vi "LogViewer.vi"(7 "Current Module(\"\" to generate an ID)":string="logViewer") -> ()   [LabVIEW 2017, in "DebugConsole.lvlib"]
uses:
  DebugConsole.lvlib
  Utility/_support/Periodic String Filter Level.ctl
  Utility/Periodic String Filter Setting.ctl
  <vilib>/addons/_JKI Toolkits/State Machine/_JKI_lib_State_Machine.llb/Parse State Queue__JKI_lib_State_Machine.vi
  _csmlite/_Engine.vi
  _csmlite/_PassAllowedMessage - MsgList.vi
  Communicable State Machine.lvlib
  _Shared/CSM Shared.lvlib
  _Support/csm-tool-support.lvlib
  _csmHelper/API with lvcsm Support/CSM-Helper API with lvcsm Support.lvlib
  addons/Logger/CSM File Logger.lvlib
  _ui/csm-ui-support.lvlib
  _csmlite/_csmlite.lvlib
panel:
  out "Error(#)":i64 caption="Error(#):"
  in  "Record.Stop":bool
  in  "Record.Start":bool
  in  "Clear":bool
  in  "BackTop":bool
  in  "Toolbar.History Length(char)":i32=50000 caption="History(char)" min=1000 max=100000000 step=1
  in  "Peroid Logs":bool
  in  "Tab":T1(tab)
  out "State History":string
  out "Error History":string
  out "Userlog History":string
  out "LogInQ":i32 caption="LogInQ:"
  out "log handling Speed(#/s)":dbl caption="log handling Speed(#/s):"
  out "LogInQ change(#/s)":dbl caption="LogInQ change(#/s):"
  out "Level":T2 caption="Level:"
  in  "Stop":bool
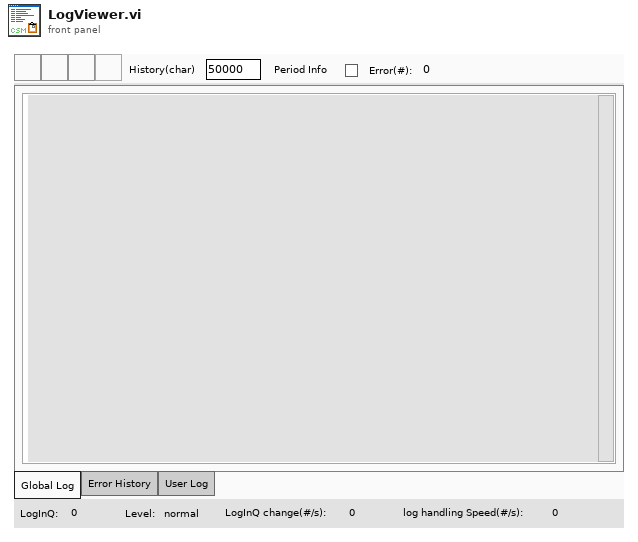
[diagram p1: front panel]
types:
  T1 = enum32{"Global Log", "Error History", "User Log"}
  T2 = typedef "Communicable State Machine.lvlib/Periodic String Filter Level.ctl" = enum16{"normal", "L1", "L2", "L3", "L4"}
  T3 = typedef "Communicable State Machine.lvlib/Periodic String Filter Setting.ctl" = cluster{"threashold(#/s)":dbl, "Check Peroid(s)":dbl}
  T4 = typedef "Communicable State Machine.lvlib/_CSM_GlobalLog_MSG.ctl" = cluster{"Name (\"\" to Use UUID)":string, "Current State":string, "Arguments":string, "Source Message":T5, "Source Module":string, "Complete(T)/Start(F)":bool, "LogType":T6, "Time Stamp":timestamp}
  T5 = typedef "Communicable State Machine.lvlib/_CSM_Response Source Message.ctl" = cluster{"‘State":string, "’Arguments":string, "’Error":errorcluster}
  T6 = typedef "Communicable State Machine.lvlib/_CSM_GlobalLog_MSG_TYPE.ctl" = enum16{"User Log", "State Change", "Status", "Interrupt", "Register", "Unregister", "Error Log", "Module Created", "Module Destroyed", "Async Message", "No-Rep Async Message", "Sync Message"}
  T7 = enum32{"Invalid", "Standard", "Closed", "Hidden", "Minimized", "Maximized"}
  T8 = enum32{"invalid app kind", "Development System", "Run Time System", "Student Edition", "Embedded LabVIEW", "Evaluation", "Custom"}
  T9 = typedef "LVPoint32TypeDef.ctl" = cluster{"Horizontal":i32, "Vertical":i32}
  T10 = cluster{"Shift":bool, "Ctrl":bool, "Alt":bool, "Cmd":bool, "Opt":bool}
  T11 = cluster{"Core":cluster{"Current VI Reference":refnum<vi>, "Close Panel on Exit?":bool}, "Toolbar.Advance":refnum<vi>[], "LoggerWatchDogQueue":refnum<queue>, "LogFile":path}
  T12 = cluster{"Current VI Reference":refnum<vi>, "Close Panel on Exit?":bool}
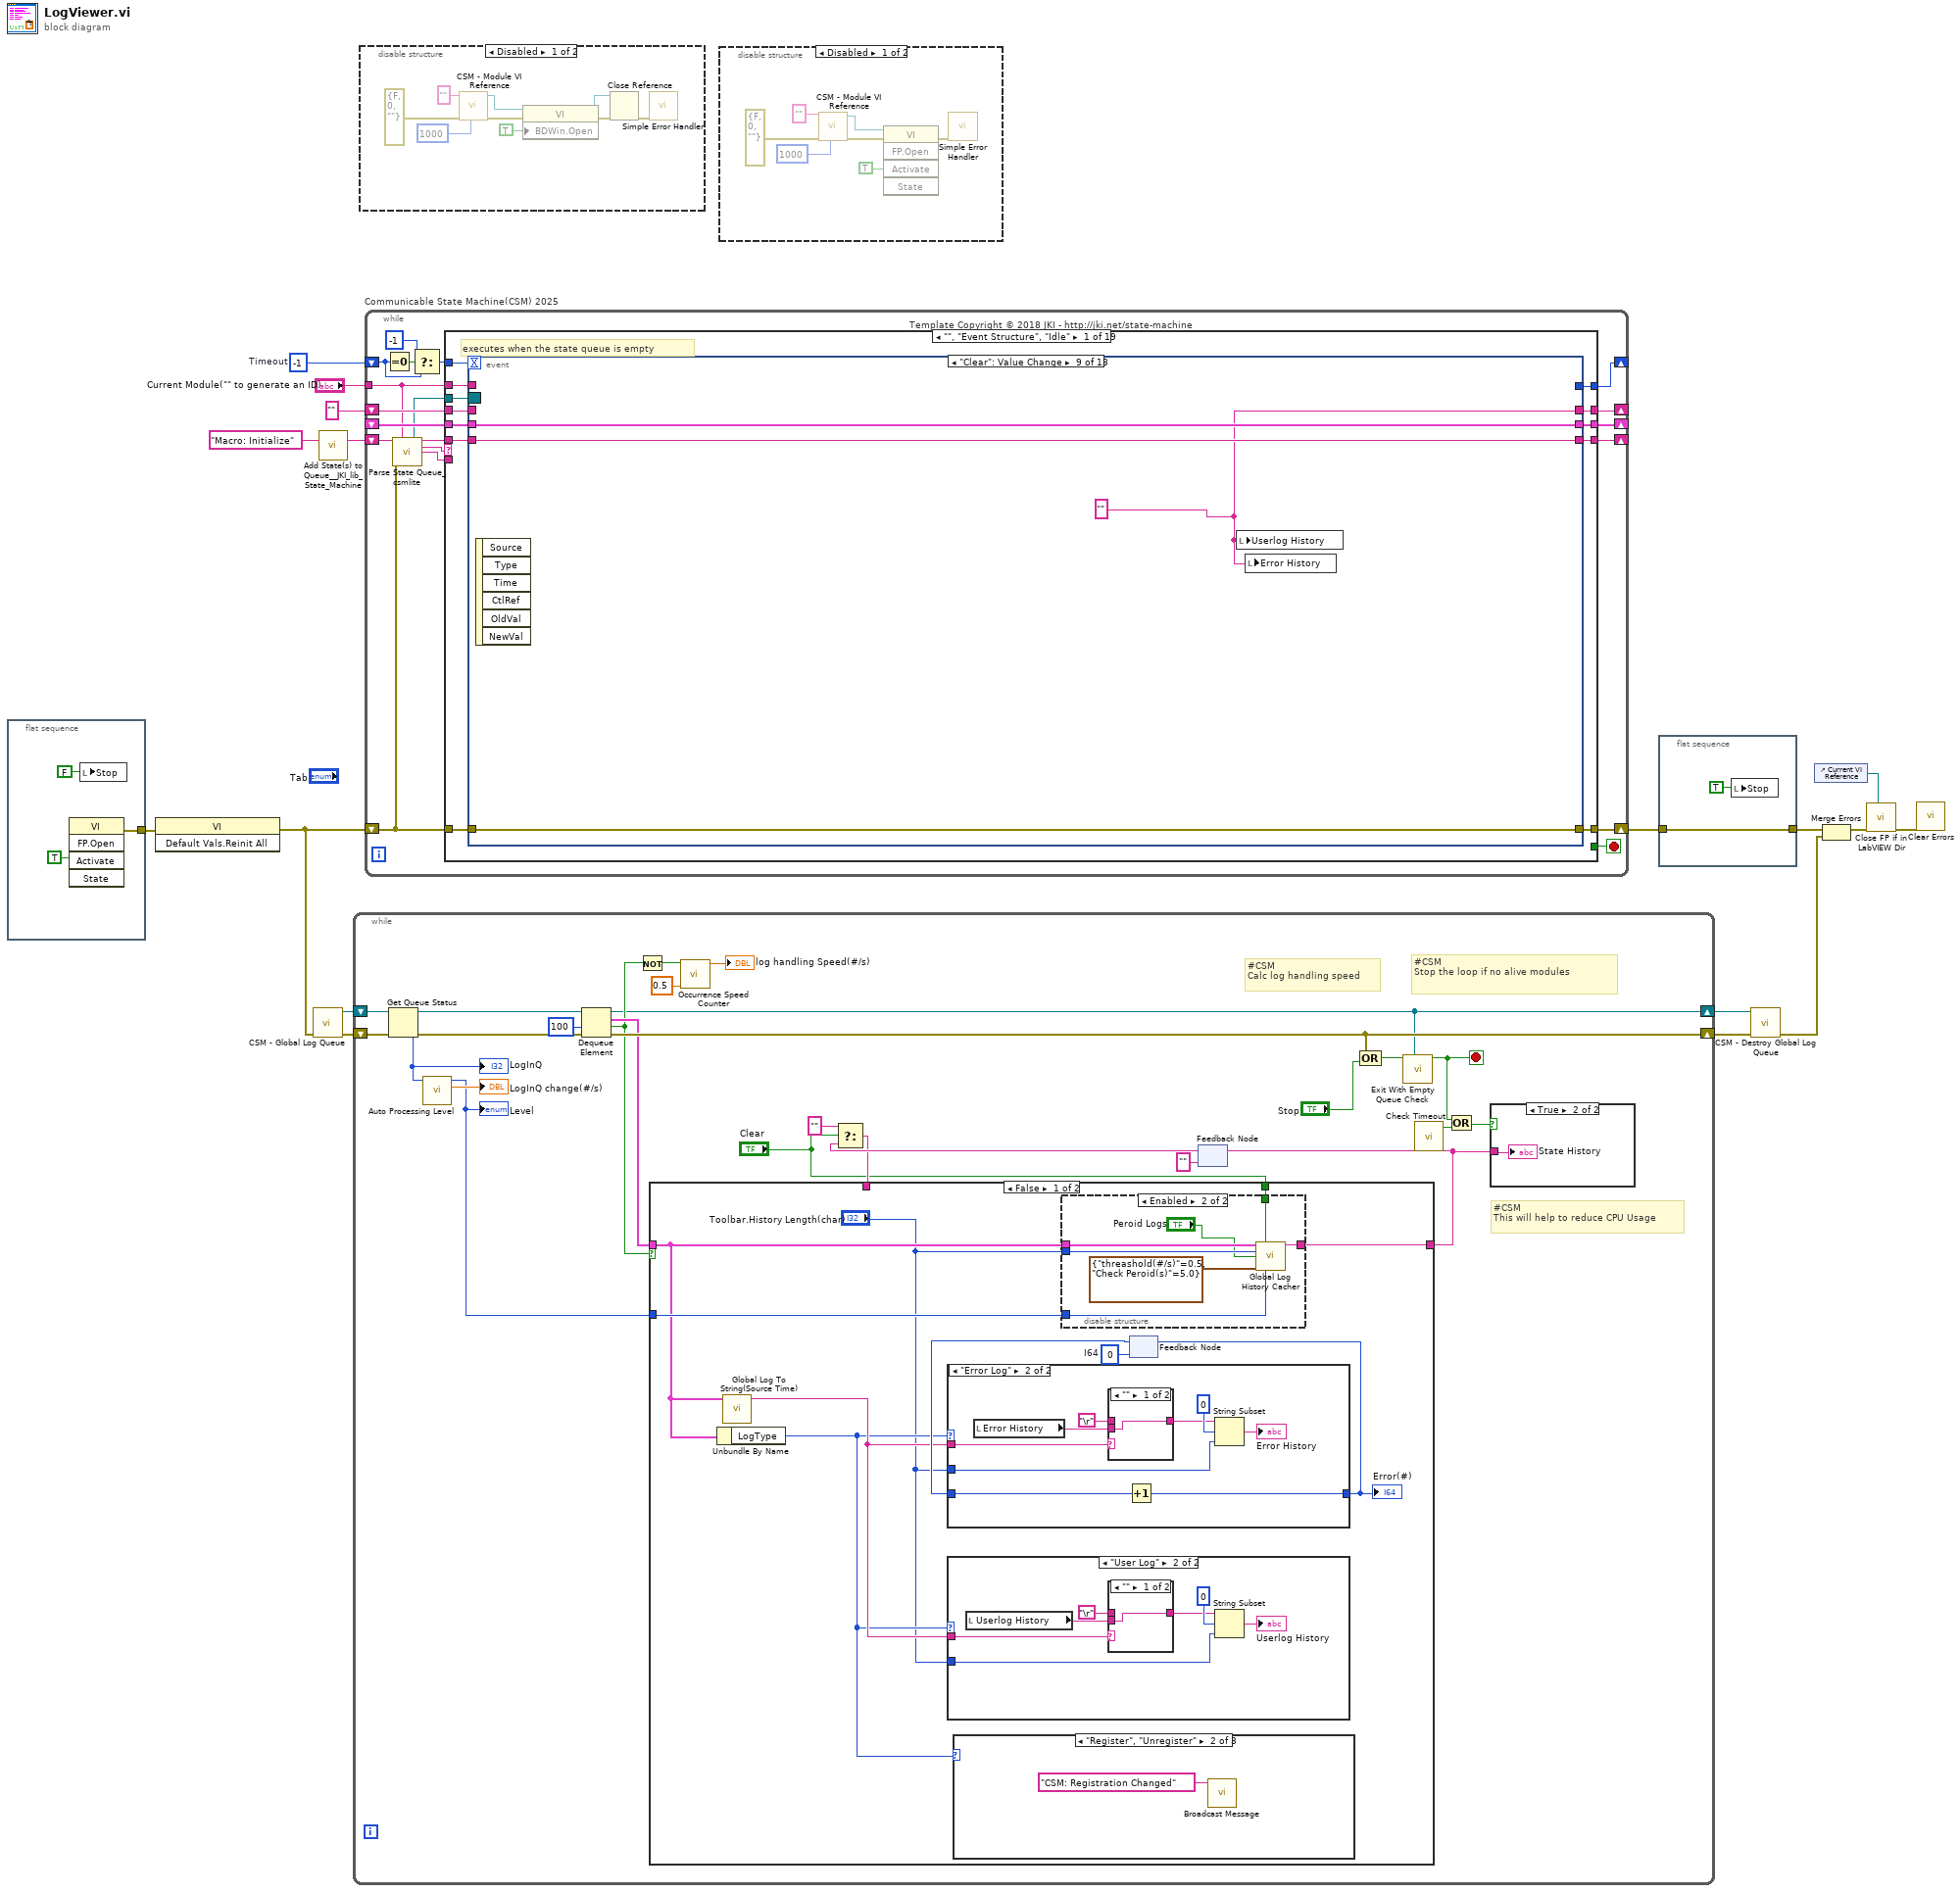
[diagram p0: block diagram]
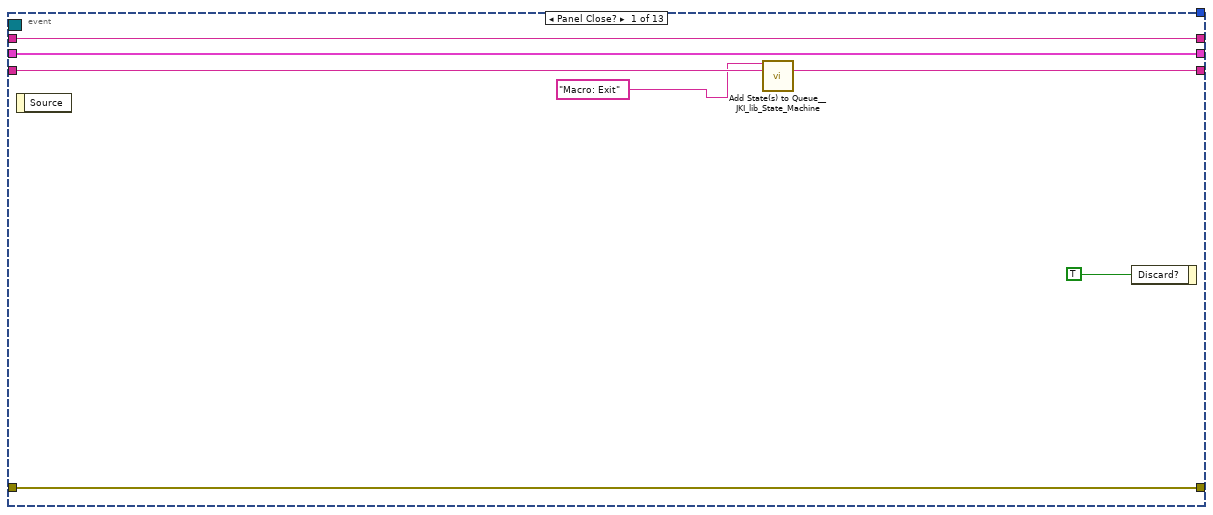
[diagram p4: hidden frame]
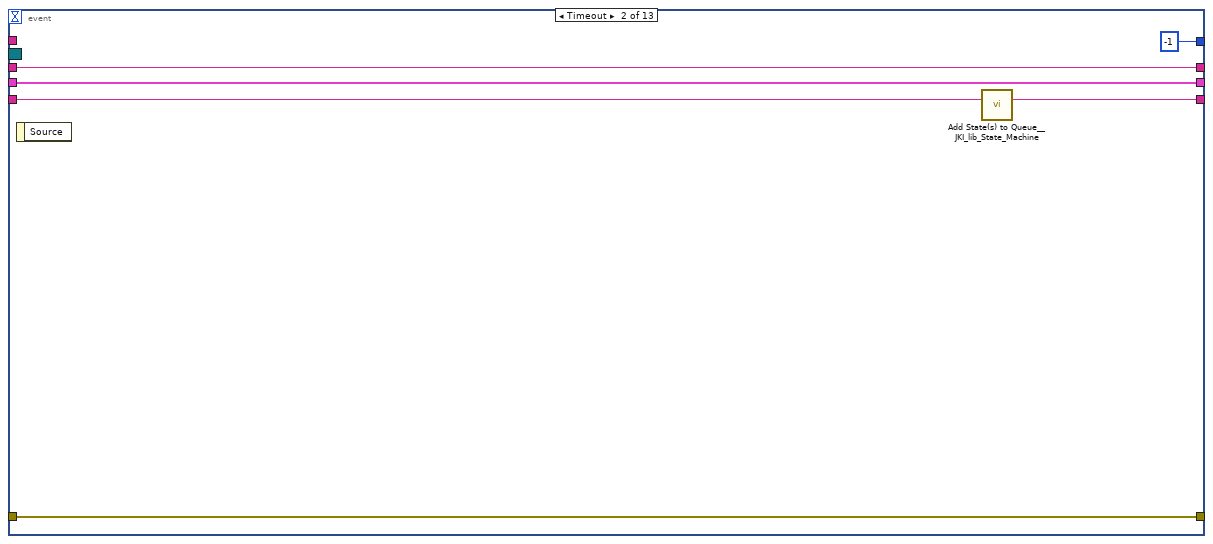
[diagram p5: hidden frame]
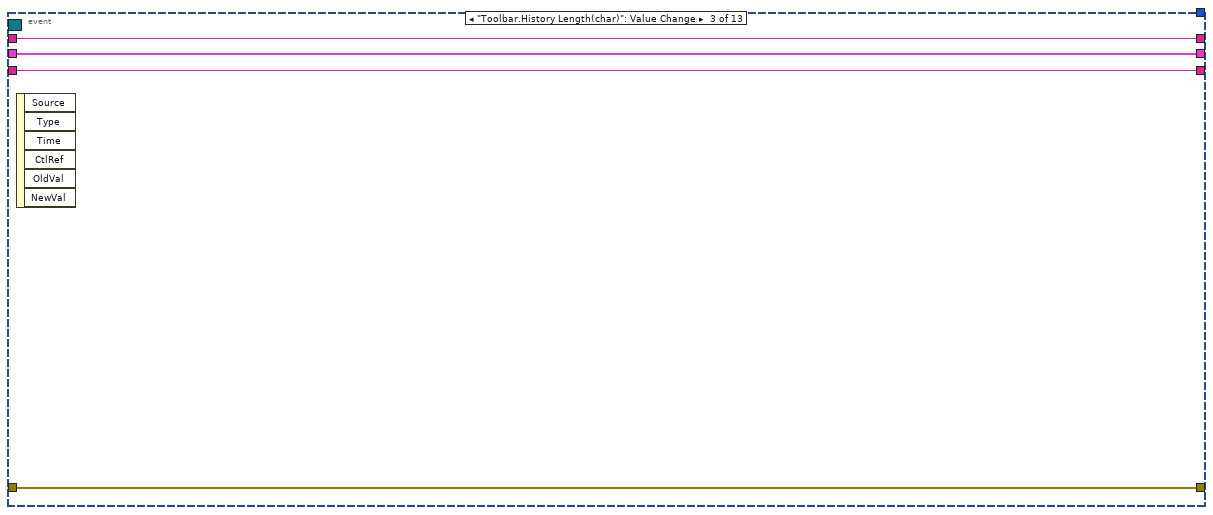
[diagram p6: hidden frame]
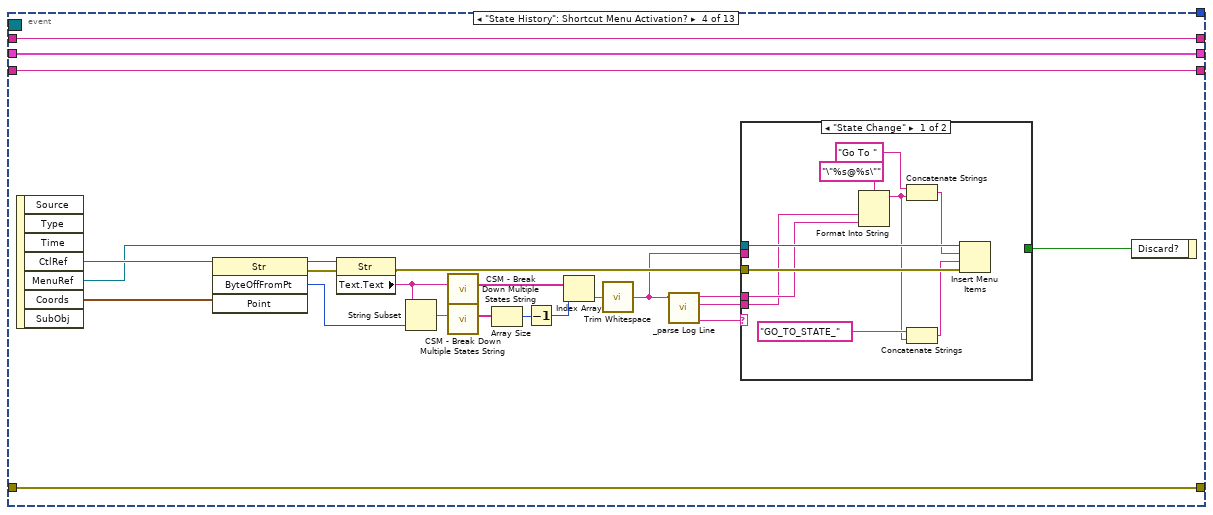
[diagram p7: hidden frame]
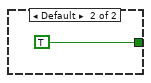
[diagram p8: hidden frame]
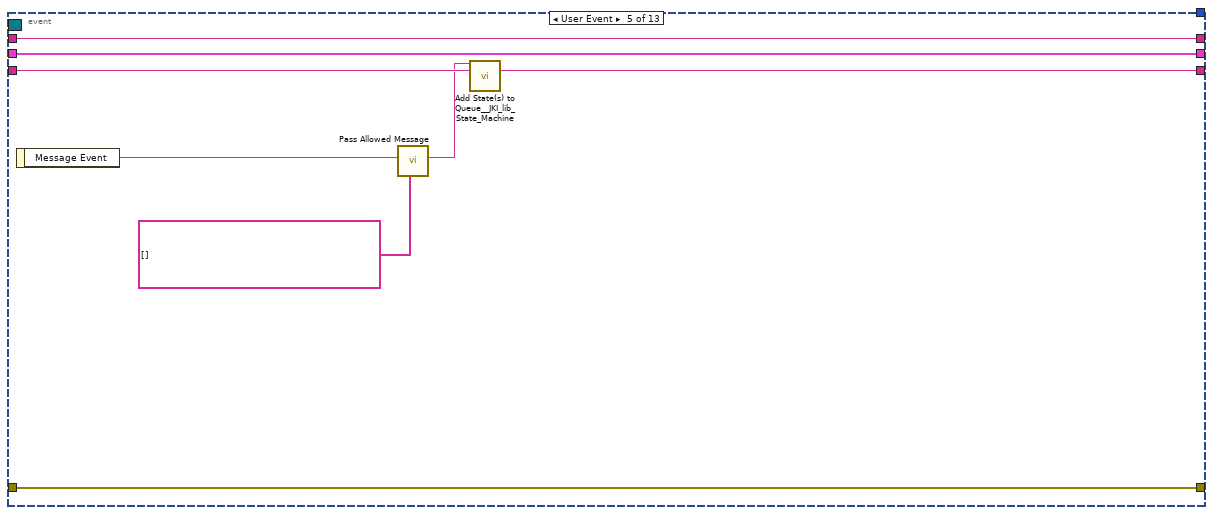
[diagram p9: hidden frame]
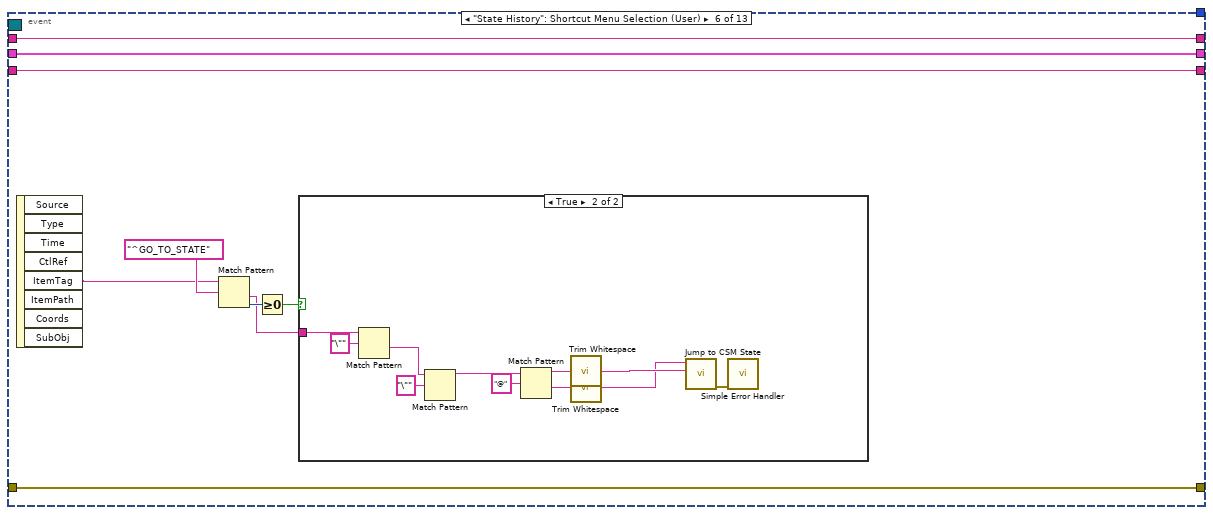
[diagram p10: hidden frame]
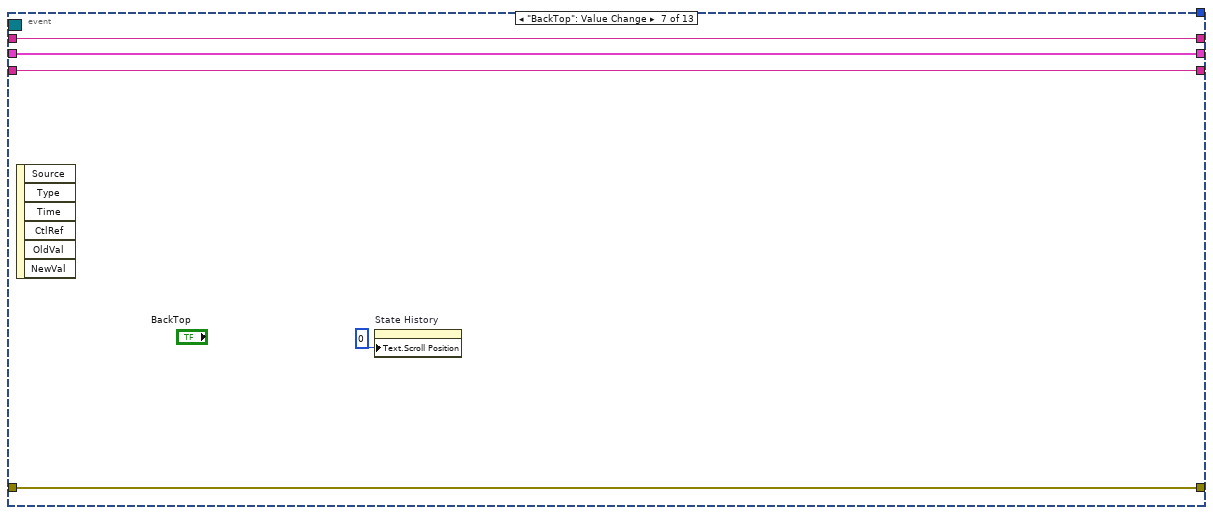
[diagram p12: hidden frame]
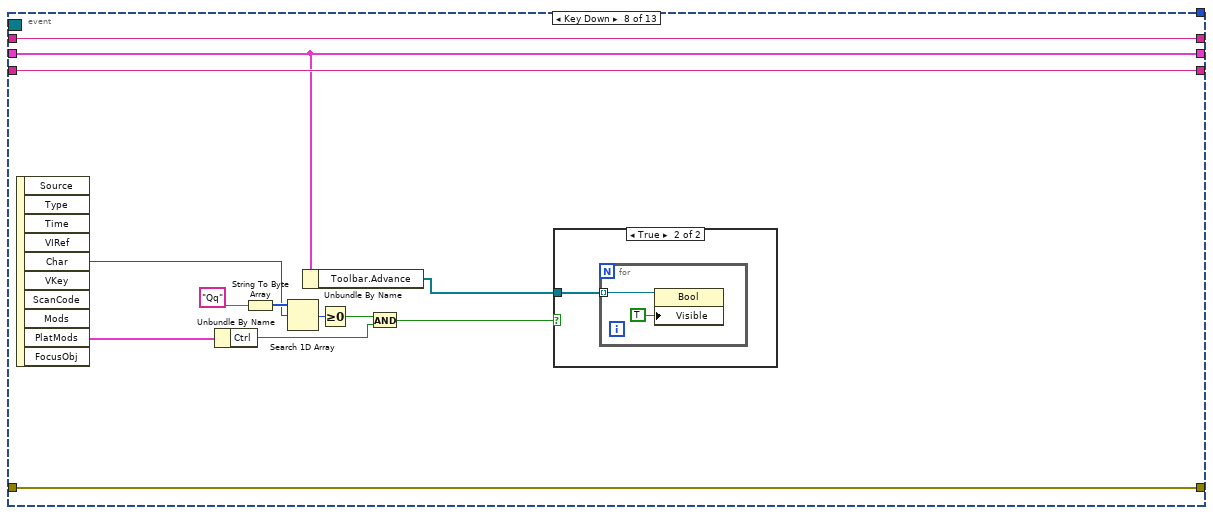
[diagram p13: hidden frame]
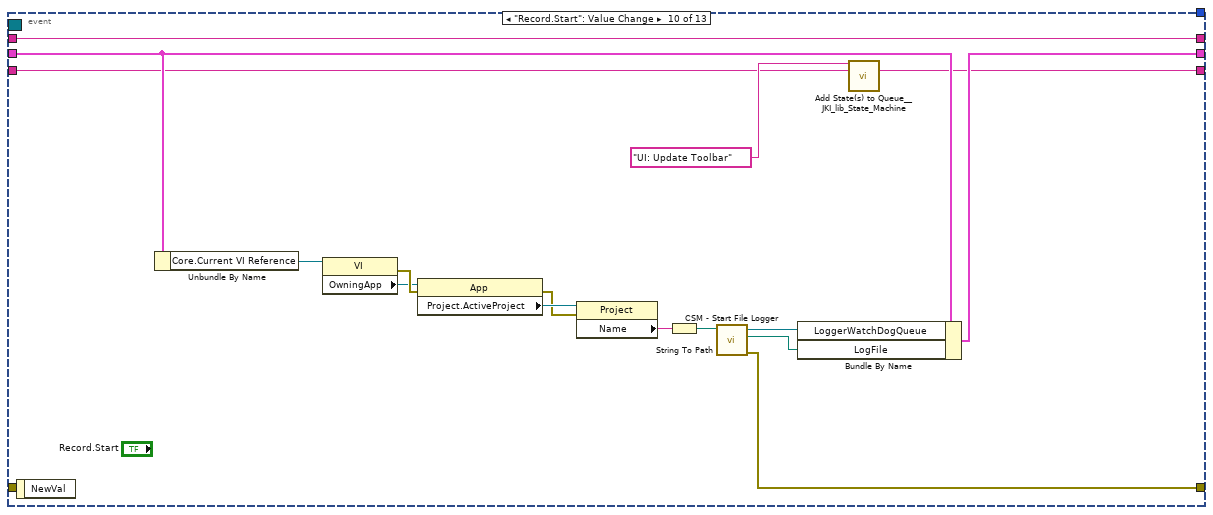
[diagram p15: hidden frame]
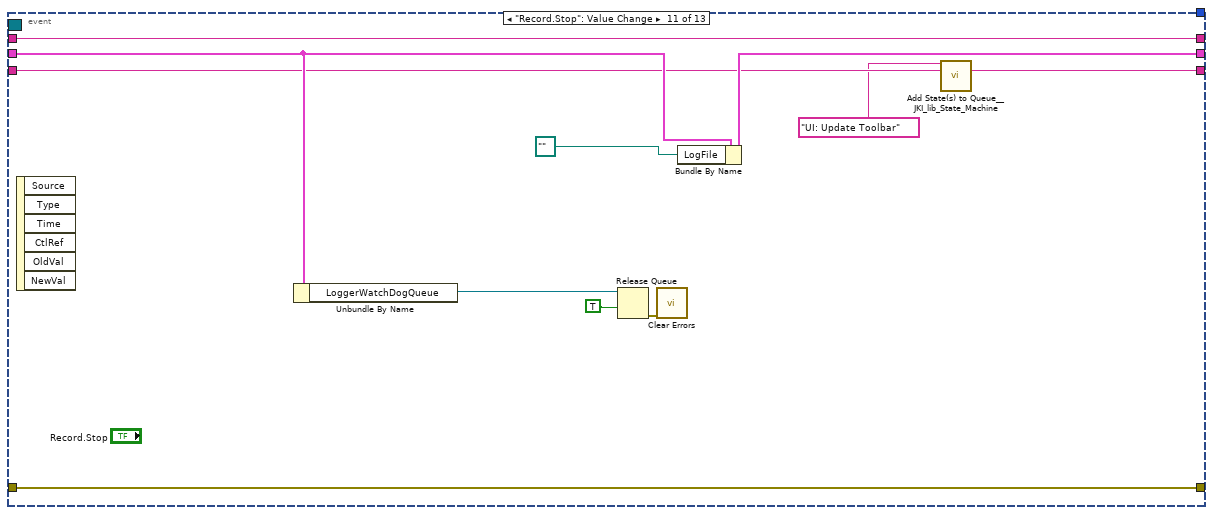
[diagram p16: hidden frame]
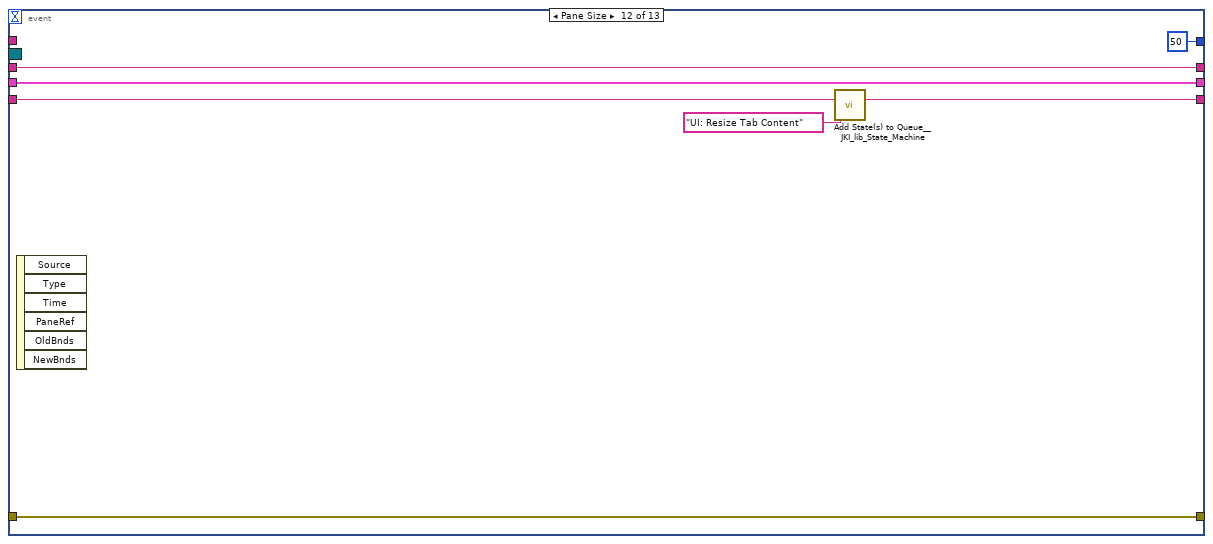
[diagram p17: hidden frame]
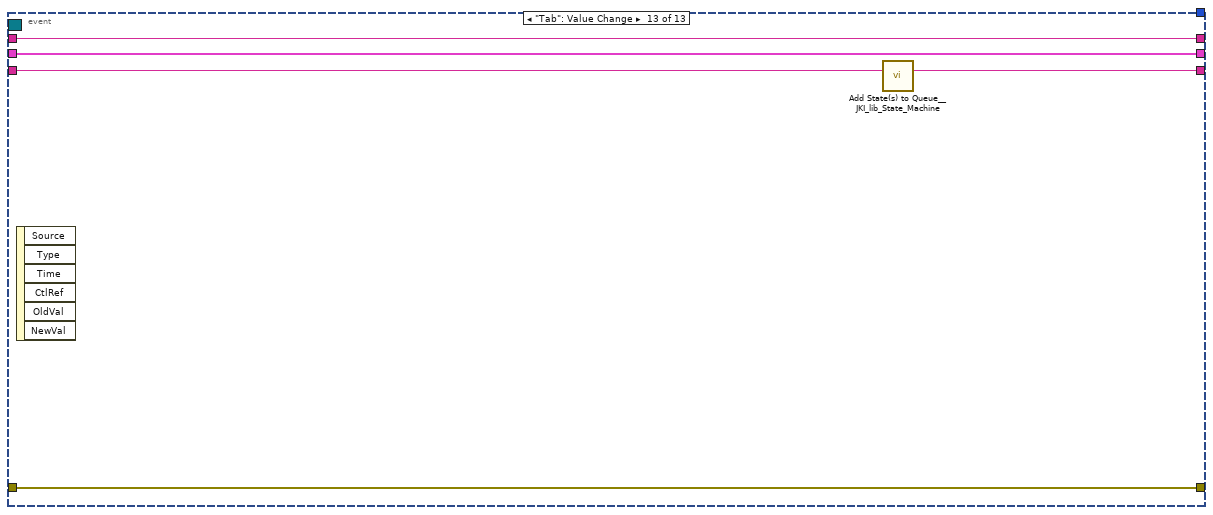
[diagram p18: hidden frame]
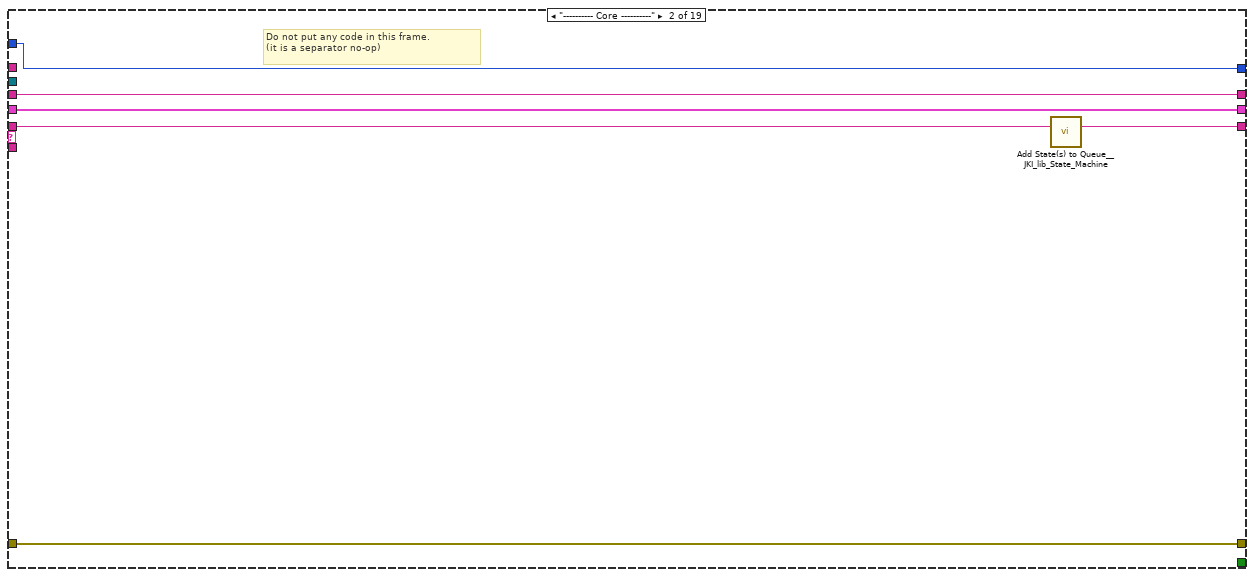
[diagram p19: hidden frame]
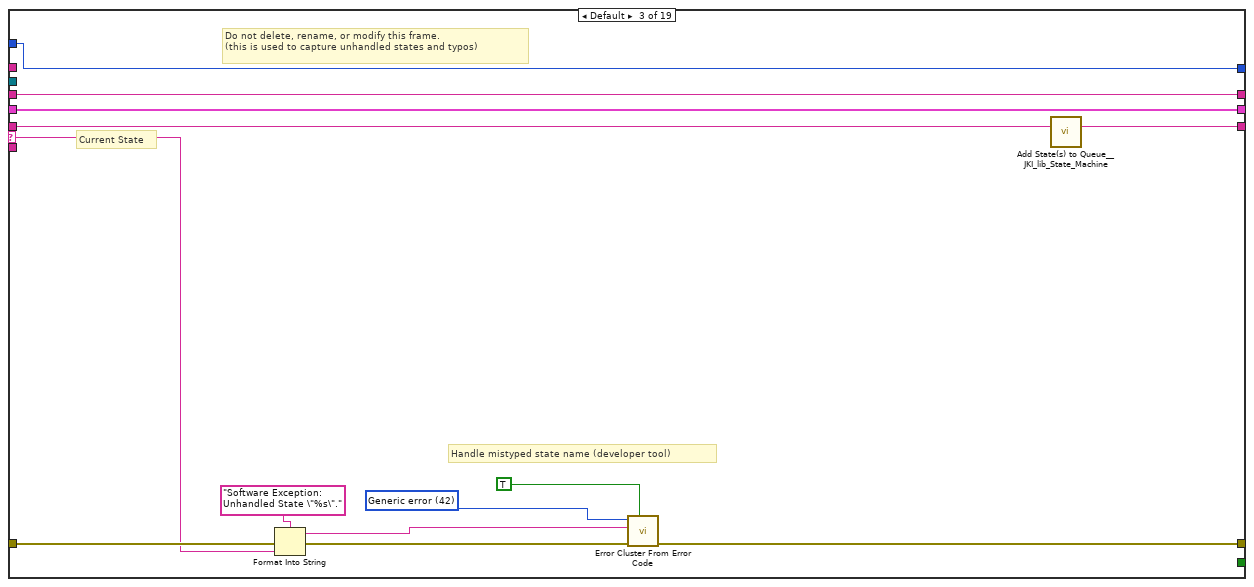
[diagram p20: hidden frame]
diagram:
  w10 = -1  # Timeout
  n1 = flat-sequence {
    tunnel: [w18] -> w6
    frame #0 {
      n2 = invoke class="VI" method="FP.Open"("Activate"=TRUE ("Activate?")) -> (error out=w18:errorcluster)  [unwired: 4 in, 4 out]
      n3 = local write "Stop"(FALSE ("Stop")) -> ()
    }
  }
  n4 = invoke class="VI" method="Default Vals.Reinit All"(error in=w6) -> (error out=w1:errorcluster)  [unwired: 2 in, 2 out]
  n5 = call "CSM - Global Log Queue.vi"("Error In"=w1) -> ("error out"=w16:errorcluster, "Global Log Queue"=w14:refnum<queue>)  [unwired: 9 in]
  n6 = call <vilib>:"Add State(s) to Queue__JKI_lib_State_Machine.vi"("State(s) in (\"\")"="Macro: Initialize") -> ("States Out"=w13:string)  [unwired: 14 in]
  n7 = while {
    shift-right: [w45] -> w17
    shift-left: w16 -> [w42]
    shift-right: [w33] -> w15
    shift-left: w14 -> [w46]
    stop <- w26 stop-if-true
    # "#CSM\nCalc log handling speed"
    # "#CSM\nStop the loop if no alive modules"
    # "#CSM\nThis will help to reduce CPU Usage"
    n8 = Get Queue Status(queue=w46, error in (no error)=w42) -> (queue out=w44:refnum<queue>, error out=w43:errorcluster, # elements in queue=w29:i32)  [unwired: 1 in, 5 out]
    "LogInQ" <- w29
    n9 = call "Auto Processing Level.vi"("#Left In Q"=w29) -> ("LogInQ Changing Speed (#/s)"=→"LogInQ change(#/s)":dbl, "Level"=w28:T2)  [unwired: 8 in, 1 out]
    "Level" <- w28
    n10 = Dequeue Element(queue=w44, timeout in ms (-1)=100, error in (no error)=w43) -> (queue out=w33:refnum<queue>, element=w41:T4, timed out?=w35:bool, error out=w45:errorcluster)
    n11 = Not(x=w35) -> (.not. x?=w34:bool)
    n12 = call "Occurrence Speed Counter.vi"("Period (0.1s)"=0.5, "Occured? (T)"=w34) -> ("Speed (#/s)"=→"log handling Speed(#/s)":dbl)  [unwired: 7 in, 2 out]
    n13 = feedback #1("" ("String Cache")) -> (w24:string)
    n14 = Select(t="", s="Clear", f=w24) -> (s? t:f=w23:string)
    n15 = case shown="False" w35 {
      tunnel: w41 -> [w54 _]
      tunnel: [w56 w96] -> w38
      tunnel: w23 -> [_ w96]
      tunnel: w28 -> [w55 _]
      tunnel: "Clear" -> [w47 _]
      frame False {
        w52 = i64 0  # I64
        n16 = Unbundle By Name(w54) -> ("LogType"=w49:T6)
        n17 = call "Global Log To String(Source Time).vi"("Log"=w54) -> ("Log String"=w50:string)  [unwired: 9 in]
        n18 = case shown="\"User Log\"" w49 {
          tunnel: w50 -> [_ w58]
          tunnel: "Toolbar.History Length(char)" -> [_ w57]
          frame Default {
          }
          frame "User Log" {
            n19 = local read "Userlog History"() -> (w62:string)
            n20 = case shown="\"\"" w58 {
              selector: w58 -> [_ w65]
              tunnel: "\r" -> [_ w68]
              tunnel: w62 -> [w64 w67]
              tunnel: [w64 w66] -> w60
              frame "" {
              }
              frame Default {
                n21 = Concatenate Strings(w65, w68, w67) -> (w66:string)
              }
            }
            n22 = String Subset(string=w60, offset (0)=0, length (rest)=w57) -> (substring=→"Userlog History":string)
          }
        }
        n23 = case shown="\"Register\", \"Unregister\"" w49 {
          frame "User Log", Default {
          }
          frame "Register", "Unregister" {
            n24 = call "Broadcast Message.vi"("Message"="CSM: Registration Changed" ("event data")) -> ()  [unwired: 10 in, 1 out]
          }
          frame "Module Created", "Module Destroyed" {
            n25 = call "Broadcast Message.vi"("Message"="CSM: Module List Changed") -> ()  [unwired: 10 in, 1 out]
          }
        }
        n26 = disable-structure shown="Enabled" {
          disable-tunnel: w54 -> [w88 w94]
          disable-tunnel: [w86 w95] -> w56
          disable-tunnel: w55 -> [_ w93]
          disable-tunnel: "Toolbar.History Length(char)" -> [_ w91]
          disable-tunnel: w47 -> [_ w89]
          frame Disabled {
            # "#CSM \nno periodical filter"
            n27 = call "Global Log To String(Source Time).vi"("Log"=w88) -> ("Log String"=w87:string)  [unwired: 9 in]
            n28 = call "String History Cacher.vi"("String"=w87) -> ("String Cache"=w86:string)  [unwired: 10 in]
          }
          frame Enabled {
            n29 = call "Global Log History Cacher.vi"("Global Log Data"=w94, "Reset?"=w89, "Length (10000)"=w91, "With Periodic Info? (T)"="Peroid Logs", "Settings"=T3 {"threashold(#/s)"=0.5, "Check Peroid(s)"=5.0}, "Level (Normal)"=w93) -> ("String Cache"=w95:string)  [unwired: 9 in]
          }
        }
        n30 = feedback #2(w52) -> (w51:i64)
        n31 = case shown="\"Error Log\"" w49 {
          tunnel: w50 -> [_ w75]
          tunnel: "Toolbar.History Length(char)" -> [_ w74]
          tunnel: [w71 w73] -> w53
          tunnel: w51 -> [w71 w72]
          frame "User Log", Default {
          }
          frame "Error Log" {
            n32 = local read "Error History"() -> (w79:string)
            n33 = case shown="\"\"" w75 {
              selector: w75 -> [_ w82]
              tunnel: "\r" -> [_ w85]
              tunnel: w79 -> [w81 w84]
              tunnel: [w81 w83] -> w77
              frame "" {
              }
              frame Default {
                n34 = Concatenate Strings(w82, w85, w84) -> (w83:string)
              }
            }
            n35 = Increment(x=w72) -> (x+1=w73:i64)
            n36 = String Subset(string=w77, offset (0)=0, length (rest)=w74) -> (substring=→"Error History":string)
          }
        }
        "Error(#)" <- w53
        n37 = feedback-in #2(w53) -> ()
      }
      frame True {
      }
    }
    n38 = feedback-in #1(w38) -> ()
    n39 = Compound Arithmetic op=OR(w45, "Stop") -> (w31:bool)
    n40 = call "Exit With Empty Queue Check.vi"("Queue"=w33, "Stop"=w31) -> ("Exit"=w26:bool)  [unwired: 8 in, 1 out]
    n41 = call "Check Timeout.vi"() -> ("Timeout"=w39:bool)  [unwired: 8 in]
    n42 = Or(x=w26, y=w39) -> (x .or. y?=w32:bool)
    n43 = case shown="True" w32 {
      tunnel: w38 -> [_ w97]
      frame False {
      }
      frame True {
        "State History" <- w97
      }
    }
  }
  n44 = disable-structure shown="Disabled" {
    frame Disabled {
      n45 = call "CSM - Module VI Reference.vi"("Response Timeout (-2 Using Global Settings)"=1000 ("Response Timeout(5000 ms)"), "error in (no error)"=errorcluster {"status"=FALSE, "code"=0, "source"=""}, "CSM Name"="") -> ("error out"=w106:errorcluster, "CSM Module VIRef"=w103:refnum<vi>)  [unwired: 7 in]
      n46 = property class="VI"(reference=w103, error in=w106, "BDWin.Open"=TRUE ("Block Diagram Window:Open")) -> (reference out=w104:refnum<vi>, error out=w105:errorcluster)
      n47 = Close Reference(reference=w104, error in (no error)=w105) -> (error out=w102:errorcluster)
      n48 = call <vilib>:"Simple Error Handler.vi"("error in (no error)"=w102) -> ()  [unwired: 4 in, 5 out]
    }
    frame Enabled {
    }
  }
  n49 = while "Communicable State Machine(CSM) 2025" {
    shift-right: [w118] -> _
    shift-left: _ -> [w117]
    shift-right: [w121] -> w7
    shift-left: w1 -> [w116]
    shift-right: [w120] -> _
    shift-left: w13 -> [w122]
    tunnel: "Current Module(\"\" to generate an ID)" -> [w108]
    shift-right: [w114] -> _
    shift-left: "" ("String Cache") -> [w115]
    shift-right: [w113] -> _
    shift-left: w10 -> [w110]
    stop <- w119 stop-if-true
    # "Template Copyright © 2018 JKI - http://jki.net/state-machine"
    n50 = Equal To 0?(x=w110) -> (x = 0?=w112:bool)
    n51 = call "Parse State Queue_csmlite.vi"("State Queue"=w122, "Current Module(\"\" to generate an ID)"=w108, "Error In (no error)"=w116) -> ("Event Registration Refnum"=w107:refnum<event-registration>, "Remaining States"=w124:string, "Current State"=w125:string, "Arguments"=w123:string)  [unwired: 9 in]
    n52 = Select(t=-1 ("Timeout"), s=w112, f=w110) -> (s? t:f=w111:i32)
    n53 = case shown="\"\", \"Event Structure\", \"Idle\"" w125 {
      selector: w125 -> [_ _ w289 _ _ _ _ _ _ _ _ _ _ _ _ _ _ _ _]
      tunnel: w124 -> [w137 w286 w293 w314 w322 w329 w335 w345 w350 w358 w364 w372 w383 w396 w480 w498 w508 w515 w523]
      tunnel: w123 -> [_ _ _ _ _ _ _ _ _ _ _ _ w378 w390 _ _ _ _ _]
      tunnel: w117 -> [w135 w283 w291 w307 w319 w327 w332 _ w349 w353 w361 w368 w381 w392 w476 w497 w505 w512 w520]
      tunnel: [w134 w284 w295 w311 errorcluster {"status"=FALSE, "code"=0, "source"=""} ("error out") w326 w333 w342 w347 w354 w362 w370 w379 w393 w481 w499 w506 w513 w521] -> w121
      tunnel: w116 -> [w133 w284 w294 w311 w318 w326 w333 w342 w347 w355 w362 w370 w380 w394 w481 w499 w506 w513 w521]
      tunnel: [w136 w285 w292 w313 w321 w328 w334 w344 w350 w357 w363 w371 w382 w395 w480 w498 w507 w514 w522] -> w120
      tunnel: [_ _ _ _ _ TRUE _ _ _ _ _ _ _ _ _ _ _ _ _] -> w119
      tunnel: [w132 w283 w291 w312 w319 w327 w332 w343 w349 w353 w361 w368 w381 w392 w476 w497 w505 w512 w520] -> w118
      tunnel: w111 -> [w131 w281 w287 w300 w315 w323 w330 w336 w346 w351 w359 w365 w376 w388 w462 w495 w503 w509 w516]
      tunnel: w107 -> [w130 _ _ _ _ _ _ _ _ _ _ _ _ _ _ _ _ _ _]
      tunnel: w108 -> [w129 _ _ _ _ _ _ _ _ _ _ _ _ _ _ _ _ _ _]
      tunnel: w115 -> [w128 w282 w288 w301 w316 w324 w331 w340 w348 w352 w360 w369 w377 w389 w479 w496 w504 w510 w517]
      tunnel: [w127 w282 w288 w301 w316 w324 w331 w340 w348 w352 w360 w369 w377 w389 w479 w496 w504 w510 w517] -> w114
      tunnel: [w126 w281 w287 w300 w315 w323 w330 w336 w346 w351 w359 w365 w376 w388 w462 w495 w503 w509 w516] -> w113
      frame "", "Event Structure", "Idle" {
        # "executes when the state queue is empty"
        n54 = event shown="[8] \"Clear\": Value Change" {
          selector: w130 -> [_ _ _ _ _ _ _ _ _ _ _ _ _]
          dyn-events: _ -> [_ _ _ _ _ _ _ _ _ _ _ _ _]
          timeout: w131 -> [_ _ _ _ _ _ _ _ _ _ _ _ _]
          tunnel: w137 -> [w144 w150 w154 w177 w192 w205 w221 w234 w241 w243 w260 w271 w276]
          tunnel: [w143 w149 w154 w177 w193 w205 w221 w234 w241 w242 w259 w272 w277] -> w136
          tunnel: w135 -> [w141 w147 w152 w175 w195 w203 w219 w224 w239 w252 w266 w274 w279]
          tunnel: [w142 w148 w153 w176 w196 w204 w220 w233 w240 w254 w268 w275 w280] -> w134
          tunnel: w133 -> [w142 w148 w153 w176 w196 w204 w220 w233 w240 _ w268 w275 w280]
          tunnel: [w141 w147 w152 w175 w195 w203 w219 w224 w239 w255 w262 w274 w279] -> w132
          tunnel: w129 -> [_ _ _ _ _ _ _ _ _ _ _ _ _]
          tunnel: w128 -> [w138 w146 w151 w174 w194 w202 w218 w232 _ w257 w267 w273 w278]
          tunnel: [w138 w146 w151 w174 w194 w202 w218 w232 w238 w257 w267 w273 w278] -> w127
          tunnel: [_ -1 ("Timeout") _ _ _ _ _ _ _ _ _ 50 ("Timeout") _] -> w126
          event Panel Close? {
            n55 = event-data() -> ()  [unwired: 1 in, 1 out]
            n56 = call <vilib>:"Add State(s) to Queue__JKI_lib_State_Machine.vi"("State(s) in Front (\"\")"="Macro: Exit", "State(s) in (\"\")"=w144) -> ("States Out"=w143:string)  [unwired: 13 in]
            n57 = event-data("Discard?"=TRUE) -> ()  [unwired: 1 in, 1 out]
          }
          event Timeout {
            n58 = event-data() -> ()  [unwired: 1 in, 1 out]
            n59 = call <vilib>:"Add State(s) to Queue__JKI_lib_State_Machine.vi"("State(s) in (\"\")"=w150) -> ("States Out"=w149:string)  [unwired: 14 in]
          }
          event "Toolbar.History Length(char)": Value Change {
            n60 = event-data() -> ()  [unwired: 1 in, 6 out]
          }
          event "State History": Shortcut Menu Activation? {
            n61 = event-data() -> ("CtlRef"=w157:refnum<vi>, "MenuRef"=w156:refnum<k9>, "Coords"=w155:T9)  [unwired: 1 in, 4 out]
            n62 = invoke class="Str" method="ByteOffFromPt"(reference=w157, "Point"=w155) -> (reference out=w173:refnum<vi>, error out=w171:errorcluster, "ByteOffFromPt"=w172:i32)  [unwired: 2 in, 1 out]
            n63 = property class="Str"(reference=w173, error in=w171) -> (error out=w163:errorcluster, "Text.Text"=w169:string)  [unwired: 1 out]
            n64 = String Subset(string=w169, length (rest)=w172) -> (substring=w170:string)  [unwired: 1 in]
            n65 = call "CSM - Break Down Multiple States String.vi"("States"=w169) -> ("Multiple States"=w168:string[])  [unwired: 10 in]
            n66 = call "CSM - Break Down Multiple States String.vi"("States"=w170) -> ("Multiple States"=w167:string[])  [unwired: 10 in]
            n67 = Array Size(array=w167) -> (size(s)=w166:i32)
            n68 = Decrement(x=w166) -> (x-1=w165:i32)
            n69 = Index Array(array=w168, index=w165) -> (element=w164:string)
            n70 = call <vilib>:"Trim Whitespace.vi"("string"=w164) -> ("trimmed string"=w162:string)  [unwired: 1 in]
            n71 = call "_parse Log Line.vi"("String"=w162) -> ("LogType"=w161:string, "State"=w159:string, "CSM"=w160:string)  [unwired: 8 in]
            n72 = case shown="\"State Change\"" w161 {
              tunnel: w156 -> [w187 _]
              tunnel: w162 -> [_ _]
              tunnel: w163 -> [w185 _]
              tunnel: [_ TRUE] -> w158
              tunnel: w160 -> [w183 _]
              tunnel: w159 -> [w182 _]
              frame "State Change" {
                n73 = Format Into String(format string="\"%s@%s\"", w182, w183) -> (resulting string=w178:string)  [unwired: 2 in, 1 out]
                n74 = Concatenate Strings("Go To " ("format string"), w178) -> (w181:string)
                n75 = Concatenate Strings("GO_TO_STATE_" ("item tags"), w178) -> (w179:string)
                n76 = Insert Menu Items(6:w185, 7:w179, 8:w181, 9:w187) -> ()  [unwired: 2 in, 3 out]
              }
              frame Default {
              }
            }
            n77 = event-data("Discard?"=w158) -> ()  [unwired: 1 in, 1 out]
          }
          event User Event {
            n78 = event-data() -> ("Message Event"=w190:string)  [unwired: 1 in]
            n79 = call-poly "Pass Allowed Message.vi"("Allowed Message"=string[] [] ("1D array"), "JKISM External Event"=w190) -> ("States"=w191:string)  [unwired: 7 in]
            n80 = call <vilib>:"Add State(s) to Queue__JKI_lib_State_Machine.vi"("State(s) in Front (\"\")"=w191, "State(s) in (\"\")"=w192) -> ("States Out"=w193:string)  [unwired: 13 in]
          }
          event "State History": Shortcut Menu Selection (User) {
            n81 = event-data() -> ("ItemTag"=w197:string)  [unwired: 1 in, 7 out]
            n82 = Match Pattern(string=w197, regular expression="^GO_TO_STATE") -> (after substring=w198:string, offset past match=w200:i32)  [unwired: 1 in, 2 out]
            n83 = Greater Or Equal To 0?(x=w200) -> (x >= 0?=w199:bool)
            n84 = case shown="True" w199 {
              tunnel: w198 -> [_ w216]
              frame False {
              }
              frame True {
                n85 = Match Pattern(string=w216, regular expression="\"") -> (after substring=w213:string)  [unwired: 1 in, 3 out]
                n86 = Match Pattern(string=w213, regular expression="\"") -> (before substring=w212:string)  [unwired: 1 in, 3 out]
                n87 = Match Pattern(string=w212, regular expression="@") -> (before substring=w210:string, after substring=w209:string)  [unwired: 1 in, 2 out]
                n88 = call <vilib>:"Trim Whitespace.vi"("string"=w210) -> ("trimmed string"=w208:string)  [unwired: 1 in]
                n89 = call <vilib>:"Trim Whitespace.vi"("string"=w209) -> ("trimmed string"=w207:string)  [unwired: 1 in]
                n90 = call "Jump to CSM State.vi"("State"=w208, "Name"=w207) -> ("error out"=w206:errorcluster)  [unwired: 9 in]
                n91 = call <vilib>:"Simple Error Handler.vi"("error in (no error)"=w206) -> ()  [unwired: 4 in, 5 out]
              }
            }
          }
          event "BackTop": Value Change {
            n92 = event-data() -> ()  [unwired: 1 in, 6 out]
            n93 = property on="State History" class="Str"("Text.Scroll Position"=u32 0) -> ()  [unwired: 2 in, 2 out]
          }
          event Key Down {
            n94 = event-data() -> ("Char"=w222:i16, "PlatMods"=w227:T10)  [unwired: 1 in, 8 out]
            n95 = Unbundle By Name(w227) -> ("Ctrl"=w226:bool)
            n96 = String To Byte Array(string="Qq") -> (unsigned byte array=w229:u8[])
            n97 = Search 1D Array(1D array=w229, element=w222) -> (index of element=w230:i32)  [unwired: 1 in]
            n98 = Unbundle By Name(w224) -> ("Toolbar.Advance"=w223:refnum<vi>[])
            n99 = Greater Or Equal To 0?(x=w230) -> (x >= 0?=w231:bool)
            n100 = And(x=w231, y=w226) -> (x .and. y?=w225:bool)
            n101 = case shown="True" w225 {
              tunnel: w223 -> [_ w235]
              frame False {
              }
              frame True {
                n102 = for {
                  tunnel: w235 -> [w237] mode=indexing
                  n103 = property class="Bool"(reference=w237, "Visible"=TRUE) -> ()  [unwired: 1 in, 2 out]
                }
              }
            }
          }
          event "Clear": Value Change {
            w238 = "" ("String Cache")
            n104 = event-data() -> ()  [unwired: 1 in, 6 out]
            n105 = local write "Userlog History"(w238) -> ()
            n106 = local write "Error History"(w238) -> ()
          }
          event "Record.Start": Value Change {
            n107 = event-data() -> ()  [unwired: 1 in, 1 out]
            n108 = Unbundle By Name(w252) -> ("Core.Current VI Reference"=w251:refnum<vi>)
            n109 = property class="VI"(reference=w251) -> (error out=w250:errorcluster, "OwningApp"=w249:refnum<vi>)  [unwired: 1 in, 1 out]
            n110 = property class="App"(reference=w249, error in=w250) -> (error out=w247:errorcluster, "Project.ActiveProject"=w248:refnum<vi>)  [unwired: 1 out]
            n111 = property class="Project"(reference=w248, error in=w247) -> ("Name"=w246:string)  [unwired: 2 out]
            n112 = String To Path(string=w246) -> (path=w245:path)
            n113 = call "CSM - Start File Logger.vi"("Log File Path"=w245) -> ("error out"=w254:errorcluster, "Log File"=w253:path, "Watchdog Queue"=w256:refnum<queue>)  [unwired: 8 in]
            n114 = Bundle By Name(cluster=w252, "LoggerWatchDogQueue"=w256, "LogFile"=w253) -> (w255:T11)
            n115 = call <vilib>:"Add State(s) to Queue__JKI_lib_State_Machine.vi"("State(s) in Front (\"\")"="UI: Update Toolbar" ("State(s) in Front (\"\")"), "State(s) in (\"\")"=w243) -> ("States Out"=w242:string)  [unwired: 13 in]
          }
          event "Record.Stop": Value Change {
            n116 = event-data() -> ()  [unwired: 1 in, 6 out]
            n117 = Unbundle By Name(w266) -> ("LoggerWatchDogQueue"=w265:refnum<queue>)
            n118 = Release Queue(queue=w265, force destroy? (F)=TRUE) -> (error out=w263:errorcluster)  [unwired: 1 in, 2 out]
            n119 = call <vilib>:"Clear Errors.vi"("error in (no error)"=w263) -> ()  [unwired: 5 in, 2 out]
            n120 = Bundle By Name(cluster=w266, "LogFile"=path "") -> (w262:T11)
            n121 = call <vilib>:"Add State(s) to Queue__JKI_lib_State_Machine.vi"("State(s) in Front (\"\")"="UI: Update Toolbar" ("State(s) in Front (\"\")"), "State(s) in (\"\")"=w260) -> ("States Out"=w259:string)  [unwired: 13 in]
          }
          event Pane Size {
            n122 = event-data() -> ()  [unwired: 1 in, 6 out]
            n123 = call <vilib>:"Add State(s) to Queue__JKI_lib_State_Machine.vi"("State(s) in (\"\")"=w271, "State(s) at Back (\"\")"="UI: Resize Tab Content" ("State(s) in Front (\"\")")) -> ("States Out"=w272:string)  [unwired: 13 in]
          }
          event "Tab": Value Change {
            n124 = event-data() -> ()  [unwired: 1 in, 6 out]
            n125 = call <vilib>:"Add State(s) to Queue__JKI_lib_State_Machine.vi"("State(s) in (\"\")"=w276) -> ("States Out"=w277:string)  [unwired: 14 in]
          }
        }
      }
      frame "---------- Core ----------" {
        # "Do not put any code in this frame.\n(it is a separator no-op)"
        n126 = call <vilib>:"Add State(s) to Queue__JKI_lib_State_Machine.vi"("State(s) in (\"\")"=w286) -> ("States Out"=w285:string)  [unwired: 14 in]
      }
      frame Default {
        w298 = 42 items=["No error", "Argument error", "Memory is full", "Out of zone", "End of file", "File already open", "Generic file I/O error", "File not found", "File permission error", "Disk is full", "Duplicate path", "Too many files open", "System feature not enabled", "Resource file not found", "Cannot add resource", "Resource not found", "Image not found", "Image memory error", "Pen does not exist", "Config type invalid", "Config token not found", "Config parse error", "Config memory error", "Bad external code format", "Bad external code offset", "External code not present", "Null window", "Destroy window error", "Null menu", "Print aborted", "Bad print record", "Print driver error", "Windows error during printing", "Memory error during printing", "Print dialog error", "Generic print error", "Invalid device refnum", "Device not found", "Device parameter error", "Device unit error", "Cannot open device", "Device call aborted", "Generic error", "Cancelled by user", "Object ID too low", "Object ID too high", "Object not in heap", "Unknown heap", "Unknown object (invalid DefProc)", "Unknown object (DefProc not in table)", "Message out of range", "Invalid (null) method", "Unknown message", "Manager call not supported", "Bad address", "Network operation in progress", "Network operation timed out", "Connection is busy", "Network attribute not supported", "Network error", "Address in use", "System out of memory", "Connection aborted", "Connection refused", "Not connected", "Already connected", "Connection closed", "Initialization error (interapplication manager)", "Bad occurrence", "Wait on unbound occurrence handler", "Occurrence queue overflow", "Datalog type conflict", "Unused", "Unrecognized type (interapplication manager)", "Memory corrupt", "Failed to make temporary DLL", "Old CIN version", "Drag socket not found", "Failed to load drop-object", "Failed to register OLE object", "Failed to release OLE object", "Format specifier type mismatch", "Unknown format specifier", "Too few format specifiers", "Too many format specifiers", "Scan failed", "Newer CIN version", "Error converting to variant", "Runtime menu error", "Password tampered", "Variant attribute not found", "Incompatible variant data type", "Event data is not available", "Event Store is not present", "Occurrence is not found", "Event Queue is not created", "Event info is not available", "Refnum passed is NULL", "Error retrieving Class GUID", "Error retrieving CoClass GUID", "Error retrieving TypeLib GUID.", "Bad built application magic bytes.", "Specific driver is different from the specific driver associated with the Logical Name.", "There is no session opened to the class driver.", "Max Error", "MAX - Error with config objects", "MAX - Error loading configuration", "MAX - Group not supported"]
        # "Current State"
        # "Do not delete, rename, or modify this frame.\n(this is used to capture unhandled states and typos)"
        # "Handle mistyped state name (developer tool)"
        n127 = Format Into String(format string="Software Exception: Unhandled State \"%s\"." ("message"), error in=w294, w289) -> (resulting string=w297:string, error out=w296:errorcluster)  [unwired: 1 in]
        n128 = call <vilib>:"Error Cluster From Error Code.vi"("show call chain? (False)"=TRUE, "error in (no error)"=w296, "error message (\"\")"=w297, "error code (0)"=w298) -> ("error out"=w295:errorcluster)  [unwired: 5 in]
        n129 = call <vilib>:"Add State(s) to Queue__JKI_lib_State_Machine.vi"("State(s) in (\"\")"=w293) -> ("States Out"=w292:string)  [unwired: 14 in]
      }
      frame "Initialize Core Data" {
        # "Do not delete, rename, or modify this frame.\n(this is used to determine panel behavior on exit)"
        # "originally closed?"
        # "exe?"
        # "If panel starts closed or is an EXE, then close it when we exit"
        n130 = property class="VI"() -> ("FP.State"=w304:T7)  [unwired: 2 in, 2 out]
        n131 = property class="App"() -> ("App.Kind"=w310:T8)  [unwired: 2 in, 2 out]
        n132 = control-ref of="Current VI Reference"() -> (w305:refnum<vi>)
        n133 = Equal?(x=w304, y=T7."Closed" ("Front Panel Window:State")) -> (x = y?=w302:bool)
        n134 = Equal?(x=w310, y=T8."Run Time System" ("Application:Kind")) -> (x = y?=w308:bool)
        n135 = Or(x=w302, y=w308) -> (x .or. y?=w306:bool)
        n136 = Bundle By Name(cluster=w307, "Core.Current VI Reference"=w305, "Core.Close Panel on Exit?"=w306) -> (w312:T11)
        n137 = call <vilib>:"Add State(s) to Queue__JKI_lib_State_Machine.vi"("State(s) in (\"\")"=w314) -> ("States Out"=w313:string)  [unwired: 14 in]
      }
      frame "Error Handler" {
        # "Unhandled Error -- Display it"
        # "Handle any errors here.\nYou can also output any states to clean-up after errors occur"
        # "Clear error"
        n138 = call <vilib>:"General Error Handler.vi"("error in (no error)"=w318) -> ()  [unwired: 10 in, 5 out]
        n139 = call <vilib>:"Add State(s) to Queue__JKI_lib_State_Machine.vi"("State(s) in Front (\"\")"="/* Post Error States", "State(s) in (\"\")"=w322) -> ("States Out"=w321:string)  [unwired: 13 in]
      }
      frame "Exit" {
        # "Do not put any code in this frame.\n(No errors that occur here will be handled.)"
        n140 = call <vilib>:"Add State(s) to Queue__JKI_lib_State_Machine.vi"("State(s) in (\"\")"=w329) -> ("States Out"=w328:string)  [unwired: 14 in]
      }
      frame "---------- Data ----------" {
        # "Do not put any code in this frame.\n(It is a separator no-op. You can make a copy of this frame to create a new Data frame)"
        n141 = call <vilib>:"Add State(s) to Queue__JKI_lib_State_Machine.vi"("State(s) in (\"\")"=w335) -> ("States Out"=w334:string)  [unwired: 14 in]
      }
      frame "Data: Initialize" {
        w337 = refnum<queue> refnum  # LoggerWatchDogQueue
        w338 = path ""  # LogFile
        w339 = refnum<vi>[] []  # Toolbar.Advance
        w341 = T12 {"Current VI Reference"=refnum, "Close Panel on Exit?"=FALSE}  # Core
        # "Data names and types of shift register data are defined by this bundle."
        # "Initialize the shift-register data, here.\n(data names are defined by what you wire into the bundle function)"
        n142 = Bundle("Core"=w341, "Toolbar.Advance"=w339, "LoggerWatchDogQueue"=w337, "LogFile"=w338) -> (w343:T11)  [unwired: 1 in]
        n143 = call <vilib>:"Add State(s) to Queue__JKI_lib_State_Machine.vi"("State(s) in (\"\")"=w345) -> ("States Out"=w344:string)  [unwired: 14 in]
      }
      frame "Data: Initialize References" {
      }
      frame "Data: Cleanup" {
        # "Cleanup any data and references, here.\n(this is called automatically, by the Macro: Exit)"
        n144 = Unbundle By Name(w353) -> ("Core.Current VI Reference"=w356:refnum<vi>)
        n145 = Close Reference(reference=w356, error in (no error)=w355) -> (error out=w354:errorcluster)
        n146 = call <vilib>:"Add State(s) to Queue__JKI_lib_State_Machine.vi"("State(s) in (\"\")"=w358) -> ("States Out"=w357:string)  [unwired: 14 in]
      }
      frame "---------- UI ----------" {
        # "Do not put any code in this frame.\n(It is a separator no-op. You can make a copy of this frame to create a new UI frame)"
        n147 = call <vilib>:"Add State(s) to Queue__JKI_lib_State_Machine.vi"("State(s) in (\"\")"=w364) -> ("States Out"=w363:string)  [unwired: 14 in]
      }
      frame "UI: Initialize" {
        # "Initialize the User Interface, here.\n(this is called automatically, by the Macro: Init)"
        n148 = Unbundle By Name(w368) -> ("Toolbar.Advance"=w367:refnum<vi>[])
        n149 = disable-structure shown="Disabled" {
          disable-tunnel: w367 -> [w373 _]
          frame Disabled {
            n150 = for {
              tunnel: w373 -> [w375] mode=indexing
              n151 = property class="Bool"(reference=w375, "Visible"=FALSE) -> ()  [unwired: 1 in, 2 out]
            }
          }
          frame Enabled {
          }
        }
        n152 = local write "Peroid Logs"(TRUE ("Filter Peroid Logs")) -> ()
        n153 = call <vilib>:"Add State(s) to Queue__JKI_lib_State_Machine.vi"("State(s) in (\"\")"=w372) -> ("States Out"=w371:string)  [unwired: 14 in]
      }
      frame "UI: Cursor Set" {
        # "Argument"
        # "Set and Unset Cursor Busy.\n(Usage: \"UI: Cursor Set >> Busy|Idle\")"
        n154 = case shown="\"Idle\", Default" w378 {
          tunnel: w380 -> [w385 w387]
          tunnel: [w384 w386] -> w379
          frame "Idle", Default {
            n155 = call <vilib>:"Unset Busy.vi"("error in (no error)"=w385) -> ("error out"=w384:errorcluster)  [unwired: 10 in]
          }
          frame "Busy" {
            n156 = call <vilib>:"Set Busy.vi"("error in (no error)"=w387) -> ("error out"=w386:errorcluster)  [unwired: 9 in, 1 out]
          }
        }
        n157 = call <vilib>:"Add State(s) to Queue__JKI_lib_State_Machine.vi"("State(s) in (\"\")"=w383) -> ("States Out"=w382:string)  [unwired: 14 in]
      }
      frame "UI: Front Panel State" {
        # "Argument"
        # "Set Front Panel Open or Closed\n(Usage: \"UI: Front Panel State >> Open|Close\")"
        n158 = Unbundle By Name(w392) -> ("Core.Current VI Reference"=w391:refnum<vi>)
        n159 = case shown="\"Minimize\", \"Minimized\"" w390 {
          tunnel: w394 -> [w402 w417 w428 w441 w454]
          tunnel: [w404 w418 w430 w443 w456] -> w393
          tunnel: w391 -> [w403 w415 w429 w442 w455]
          frame "Open", "Standard", Default {
            w397 = T7."Standard" ("State")
            n160 = property class="VI"(reference=w403, error in=w402) -> (reference out=w400:refnum<vi>, error out=w401:errorcluster, "FP.State"=w399:T7)
            n161 = Not Equal?(x=w399, y=w397) -> (x != y?=w398:bool)
            n162 = case shown="True" w398 {
              tunnel: [w408 w410] -> w404
              tunnel: w401 -> [w407 w410]
              tunnel: w400 -> [w406 _]
              tunnel: w397 -> [w405 _]
              frame True {
                n163 = invoke class="VI" method="FP.Open"(reference=w406, error in=w407, "Activate"=TRUE, "State"=w405) -> (error out=w408:errorcluster)  [unwired: 1 in, 4 out]
              }
              frame False {
              }
            }
          }
          frame "Close", "Closed" {
            n164 = property class="VI"(reference=w415, error in=w417) -> (reference out=w414:refnum<vi>, error out=w416:errorcluster, "FP.State"=w412:T7)
            n165 = Not Equal?(x=w412, y=T7."Closed" ("Front Panel Window:State")) -> (x != y?=w411:bool)
            n166 = case shown="True" w411 {
              tunnel: [w419 w422] -> w418
              tunnel: w416 -> [w419 w421]
              tunnel: w414 -> [_ w420]
              frame False {
              }
              frame True {
                n167 = invoke class="VI" method="FP.Close"(reference=w420, error in=w421) -> (error out=w422:errorcluster)  [unwired: 1 in, 2 out]
              }
            }
          }
          frame "Hidden", "Hide" {
            w423 = T7."Hidden" ("State")
            n168 = property class="VI"(reference=w429, error in=w428) -> (reference out=w426:refnum<vi>, error out=w427:errorcluster, "FP.State"=w425:T7)
            n169 = Not Equal?(x=w425, y=w423) -> (x != y?=w424:bool)
            n170 = case shown="True" w424 {
              tunnel: [w434 w435] -> w430
              tunnel: w427 -> [w433 w435]
              tunnel: w426 -> [w432 _]
              tunnel: w423 -> [w431 _]
              frame True {
                n171 = invoke class="VI" method="FP.Open"(reference=w432, error in=w433, "State"=w431) -> (error out=w434:errorcluster)  [unwired: 2 in, 4 out]
              }
              frame False {
              }
            }
          }
          frame "Minimize", "Minimized" {
            w436 = T7."Minimized" ("State")
            n172 = property class="VI"(reference=w442, error in=w441) -> (reference out=w439:refnum<vi>, error out=w440:errorcluster, "FP.State"=w438:T7)
            n173 = Not Equal?(x=w438, y=w436) -> (x != y?=w437:bool)
            n174 = case shown="True" w437 {
              tunnel: [w447 w448] -> w443
              tunnel: w440 -> [w446 w448]
              tunnel: w439 -> [w445 _]
              tunnel: w436 -> [w444 _]
              frame True {
                n175 = invoke class="VI" method="FP.Open"(reference=w445, error in=w446, "State"=w444) -> (error out=w447:errorcluster)  [unwired: 2 in, 4 out]
              }
              frame False {
              }
            }
          }
          frame "Maximize", "Maximized" {
            w449 = T7."Maximized" ("State")
            n176 = property class="VI"(reference=w455, error in=w454) -> (reference out=w452:refnum<vi>, error out=w453:errorcluster, "FP.State"=w451:T7)
            n177 = Not Equal?(x=w451, y=w449) -> (x != y?=w450:bool)
            n178 = case shown="True" w450 {
              tunnel: [w460 w461] -> w456
              tunnel: w453 -> [w459 w461]
              tunnel: w452 -> [w458 _]
              tunnel: w449 -> [w457 _]
              frame True {
                n179 = invoke class="VI" method="FP.Open"(reference=w458, error in=w459, "State"=w457) -> (error out=w460:errorcluster)  [unwired: 2 in, 4 out]
              }
              frame False {
              }
            }
          }
        }
        n180 = call <vilib>:"Add State(s) to Queue__JKI_lib_State_Machine.vi"("State(s) in (\"\")"=w396) -> ("States Out"=w395:string)  [unwired: 14 in]
      }
      frame "UI: Update Toolbar" {
        w470 = i16 2 ("x")
        n181 = control-ref of="Record.Start"() -> (w478:refnum<vi>)
        n182 = control-ref of="Record.Stop"() -> (w477:refnum<vi>)
        n183 = Unbundle By Name(w476) -> ("Core.Current VI Reference"=w467:refnum<vi>, "LogFile"=w464:path, "LoggerWatchDogQueue"=w475:refnum<queue>)
        n184 = Not A Number/Path/Refnum?(number/path/refnum=w475) -> (NaN/Path/Refnum?=w468:bool)
        n185 = Not(x=w468) -> (.not. x?=w469:bool)
        n186 = Boolean To (0,1)(Boolean=w469) -> (0, 1=w474:i16)
        n187 = Boolean To (0,1)(Boolean=w468) -> (0, 1=w473:i16)
        n188 = Multiply(x=w470, y=w473) -> (x*y=w471:i16)
        n189 = Multiply(x=w470, y=w474) -> (x*y=w472:i16)
        n190 = Empty String/Path?(string/path=w464) -> (empty?=w463:bool)
        n191 = property class="Bool"(reference=w478, "DisabledEnum"=w472) -> ()  [unwired: 1 in, 2 out]
        n192 = property class="Bool"(reference=w477, "DisabledEnum"=w471) -> ()  [unwired: 1 in, 2 out]
        n193 = case shown="True" w463 {
          tunnel: "Running Log Viewer (CSM)" ("Front Panel Window:Title") -> [w486 w487]
          tunnel: [w485 w487] -> w465
          tunnel: w464 -> [w482 _]
          frame False {
            n194 = Path To String(path=w482) -> (string=w483:string)
            n195 = Concatenate Strings(w486, " - " ("string"), w483) -> (w485:string)
          }
          frame True {
          }
        }
        n196 = property class="VI"(reference=w467, "Front Panel.Title"=w465) -> ()  [unwired: 1 in, 2 out]
      }
      frame "UI: Resize Tab Content" {
        n197 = control-ref of="Tab"() -> (w494:refnum<vi>)
        n198 = control-ref of="Error History"() -> (w493:refnum<vi>)
        n199 = control-ref of="State History"() -> (w492:refnum<vi>)
        n200 = control-ref of="Userlog History"() -> (w488:refnum<vi>)
        n201 = invoke class="TabCtl (strict)" method="FitControlToPane"(reference=w494) -> (reference out=w491:refnum<vi>, error out=w489:errorcluster)  [unwired: 2 in, 1 out]
        n202 = Build Array(w488, w493, w492) -> (w490:refnum<vi>[])
        n203 = for {
          tunnel: w491 -> [w502]
          tunnel: w490 -> [w501] mode=indexing
          tunnel: w489 -> [w500]
          n204 = call "Fit Control to Tab.vi"("Control"=w501, "error in (no error)"=w500, "TabRef"=w502) -> ()  [unwired: 5 in, 2 out]
        }
      }
      frame "---------- Macro ----------" {
        # "Do not put any code in this frame.\n(It is a separator no-op. You can make a copy of this frame to create a new Macro frame)"
        n205 = call <vilib>:"Add State(s) to Queue__JKI_lib_State_Machine.vi"("State(s) in (\"\")"=w508) -> ("States Out"=w507:string)  [unwired: 14 in]
      }
      frame "Macro: Initialize" {
        w511 = "Data: Initialize\nData: Initialize References\nInitialize Core Data\nUI: Initialize\nUI: Front Panel State >> Open\nUI: Resize Tab Content\nUI: Update Toolbar"  # Data: Initialize Data: Initialize References Initialize Core Data UI: Initialize UI: Front Panel State >> Open UI: Resize Tab Content UI: Update Toolbar
        # "Initialization Macro\n(This is called once, when the VI starts)"
        n206 = call <vilib>:"Add State(s) to Queue__JKI_lib_State_Machine.vi"("State(s) in Front (\"\")"=w511, "State(s) in (\"\")"=w515) -> ("States Out"=w514:string)  [unwired: 13 in]
      }
      frame "Macro: Exit" {
        (unwired) ""
        # "Exit Macro\n(This is called once, when the VI exits)"
        n207 = Unbundle By Name(w520) -> ()  [unwired: 1 out]
        n208 = call <vilib>:"Add State(s) to Queue__JKI_lib_State_Machine.vi"("State(s) at Back (\"\")"="Data: Cleanup\nExit") -> ("States Out"=w518:string)  [unwired: 14 in]
        n209 = call <vilib>:"Add State(s) to Queue__JKI_lib_State_Machine.vi"("State(s) in Front (\"\")"=w518, "State(s) in (\"\")"=w523) -> ("States Out"=w522:string)  [unwired: 13 in]
      }
    }
  }
  n210 = disable-structure shown="Disabled" {
    frame Disabled {
      n211 = call "CSM - Module VI Reference.vi"("Response Timeout (-2 Using Global Settings)"=1000 ("Response Timeout(5000 ms)"), "error in (no error)"=errorcluster {"status"=FALSE, "code"=0, "source"=""}, "CSM Name"="") -> ("error out"=w530:errorcluster, "CSM Module VIRef"=w529:refnum<vi>)  [unwired: 7 in]
      n212 = invoke on="Invoke Node" class="VI" method="FP.Open"(reference=w529, error in=w530, "Activate"=TRUE ("Activate?")) -> (error out=w528:errorcluster)  [unwired: 2 in, 4 out]
      n213 = call <vilib>:"Simple Error Handler.vi"("error in (no error)"=w528) -> ()  [unwired: 4 in, 5 out]
    }
    frame Enabled {
    }
  }
  n214 = flat-sequence {
    tunnel: [w532] -> w8
    tunnel: w7 -> [w532]
    frame #0 {
      n215 = local write "Stop"(TRUE ("Stop")) -> ()
    }
  }
  n216 = call "CSM - Destroy Global Log Queue.vi"("Error In"=w17, "Global Log Queue"=w15) -> ("error out"=w9:errorcluster)  [unwired: 9 in]
  n217 = control-ref of="Current VI Reference"() -> (w4:refnum<vi>)
  n218 = Merge Errors(w8, w9) -> (w2:errorcluster)
  n219 = call "Close FP if in LabVIEW Dir.vi"("VI Refnum"=w4, "Error in"=w2) -> ("Error out"=w5:errorcluster)  [unwired: 9 in]
  n220 = call <vilib>:"Clear Errors.vi"("error in (no error)"=w5) -> ()  [unwired: 5 in, 2 out]
